vi "Init_HTTP.vi"(6 "verify server(true)":bool=TRUE, 8 "error in (no error)":errorcluster, 11 "ByteRESTBase in":refnum<class "RESTBase.lvclass">) -> (0 "error out":errorcluster, 3 "ByteRESTBase out":refnum<class "RESTBase.lvclass">)   [LabVIEW 2019, in "ByteREST.lvlib" / "RESTBase.lvclass"]
doc: "Apre una nuova connessione HTTP e setta il content type a \"application/json\""
uses:
  RESTBase.lvclass
  RESTBase.lvclass/RESTBase.ctl
  <vilib>/httpClient/LabVIEWHTTPClient.lvlib
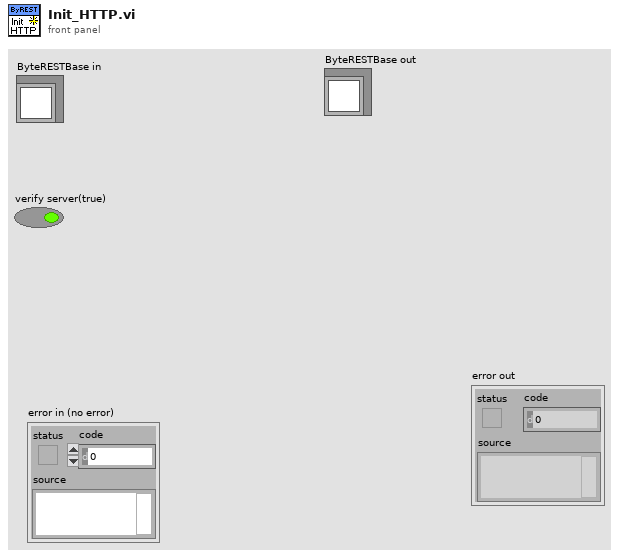
[diagram p1: front panel]
types:
  T1 = typedef "LabVIEWHTTPClient.lvlib/ClientHandle.ctl" = refnum<k1>
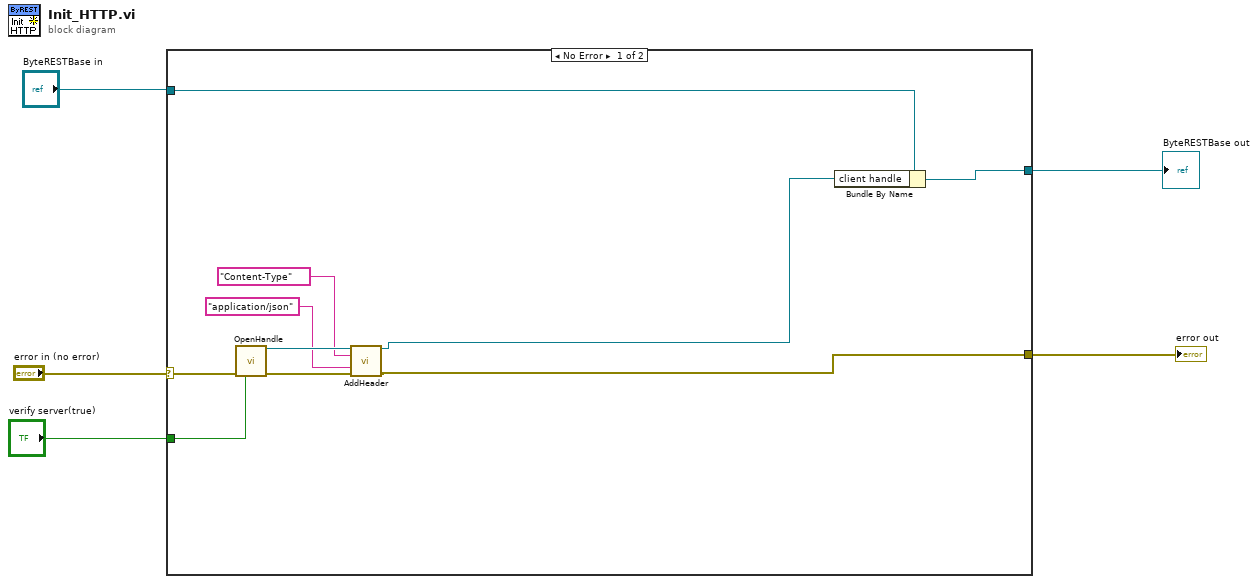
[diagram p0: block diagram]
diagram:
  n1 = case shown="No Error" "error in (no error)" {
    selector: "error in (no error)" -> [w10 w17]
    tunnel: [w7 w17] -> w4
    tunnel: [w11 w16] -> w2
    tunnel: "ByteRESTBase in" -> [w9 w16]
    tunnel: "verify server(true)" -> [w6 _]
    frame No Error {
      n2 = call <vilib>:"OpenHandle.vi"("error in (no error)"=w10, "verify server(true)"=w6) -> ("client handle out"=w14:T1, "error out"=w15:errorcluster)  [unwired: 12 in]
      n3 = call <vilib>:"AddHeader.vi"("client handle"=w14, "header"="Content-Type", "value"="application/json", "error in (no error)"=w15) -> ("client handle out"=w8:T1, "error out"=w7:errorcluster)  [unwired: 10 in]
      n4 = Bundle By Name(cluster=w9, "client handle"=w8) -> (w11:refnum<class "RESTBase.lvclass">)
    }
    frame Error {
    }
  }
  "error out" <- w4
  "ByteRESTBase out" <- w2
